vi "AreWeInTransitionTest.vi"() -> (3 "Were there any errors at all?":bool)   [LabVIEW 2013]
uses:
  Data/TypeDefs/Sailing Regimes.ctl
panel:
  out "Actual output booleans":bool[](array[boolean])
  in  "Expected output booleans":bool[](array[boolean])=[TRUE, TRUE, TRUE, TRUE, TRUE, TRUE]
  in  "Regime inputs":T1[](array[typedef])=[enum."Tack - Bow across wind", enum."Turn between Upwind/Reach - Starboard Tack", enum."Turn between Reach/Run - Starboard Tack", enum."Jibe - Stern across wind", enum."Turn between Reach/Run - Port Tack", enum."Turn between Upwind/Reach - Port Tack", enum."Reach - Starboard Tack", enum."Reach - Port Tack"]
  out "Are chosen regimes right?":bool[](array[boolean])=[TRUE, TRUE, TRUE, TRUE, TRUE, TRUE]
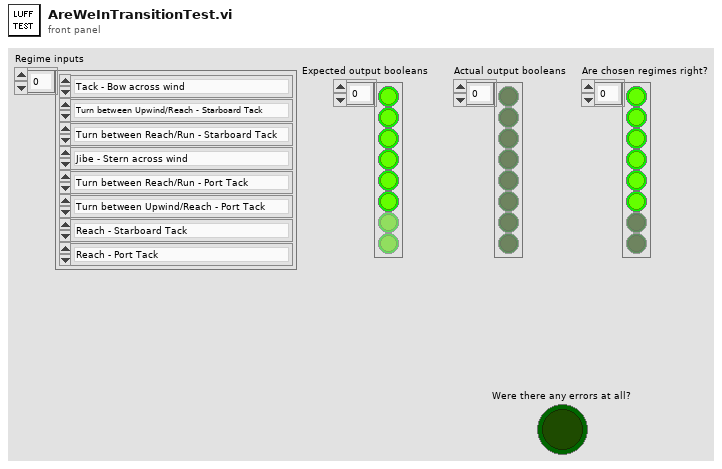
[diagram p1: front panel]
types:
  T1 = typedef "Sailing Regimes.ctl" = enum16{"Tack - Bow across wind", "Upwind - Starboard Tack", "Turn between Upwind/Reach - Starboard Tack", "Reach - Starboard Tack", "Turn between Reach/Run - Starboard Tack", "Run - Starboard Tack", "Jibe - Stern across wind", "Run - Port Tack", "Turn between Reach/Run - Port Tack", "Reach - Port Tack", "Turn between Upwind/Reach - Port Tack", "Upwind - Port Tack"}
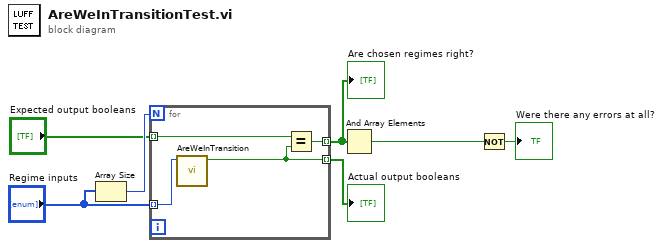
[diagram p0: block diagram]
diagram:
  n1 = Array Size(array="Regime inputs") -> (size(s)=w7:i32)
  n2 = for {
    N: w7 -> [_]
    tunnel: "Expected output booleans" -> [w11] mode=indexing
    tunnel: [w10] -> w6 mode=indexing
    tunnel: "Regime inputs" -> [w9] mode=indexing
    tunnel: [w8] -> w1 mode=indexing
    n3 = call "AreWeInTransition.vi"("Last Commanded Sailing Regime"=w9) -> ("Are We In Transition?"=w8:bool)  [unwired: 10 in]
    n4 = Equal?(x=w11, y=w8) -> (x = y?=w10:bool)
  }
  "Are chosen regimes right?" <- w6
  "Actual output booleans" <- w1
  n5 = And Array Elements(Boolean array=w6) -> (logical AND=w4:bool)
  n6 = Not(x=w4) -> (.not. x?=→"Were there any errors at all?":bool)
